vi "HostFormatPacket (1).vi"(11 "Enum in":u8) -> (3 "data string":string)   [LabVIEW 2017]
uses:
  Sensors/DataStreamIndex.ctl
  HostDataGLOBAL.vi
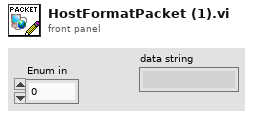
[diagram p1: front panel]
types:
  T1 = typedef "DataStreamIndex.ctl" = enum16{"SuspensionPT (PSI)", "MagBrakePT (PSI)", "Baby HPPT (PSI)", "BigRight HPPT (PSI)", "BigLeft HPPT (PSI)", "HallEffect FrontLeft (V)", "HallEffect FrontRight (V)", "HallEffect BackRight (V)", "HallEffect BackLeft (V)", "LinearPot FrontRight (V)", "LinearPot FrontLeft (V)", "LinearPot BackRight (V)", "LinearPot BackLeft (V)", "Speed (m/s)", "Distance (m)", "Piezo (V)", "Battery Voltage (V)", "Battery Current", "Battery Temperature (C)", "cRIO Temperature (C)", "Right Big Tank Temperature (C)", "Left Big Tank Temperature (C)", "Baby Tank Temperature (C)", "Right Manifold Temperature (C)", "Left Manifold Temperature (C)", "IMU Acceleration (m/s2)", "IMU Pressure (Pa)", "IMU Temperature (C)"}
  T2 = cluster{"Team ID":u8, "Enum in":u8, u32, u32, u32, u32, u32, u32, u32, u32}
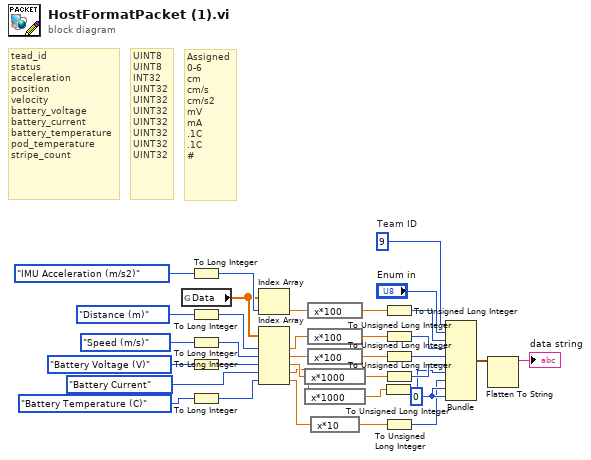
[diagram p0: block diagram]
diagram:
  w33 = u32 0
  w25 = u8 9  # Team ID
  # "Assigned\n0-6\ncm\ncm/s\ncm/s2\nmV\nmA\n.1C\n.1C\n#"
  # "UINT8\nUINT8\nINT32\nUINT32\nUINT32\nUINT32\nUINT32\nUINT32\nUINT32\nUINT32"
  # "tead_id\nstatus\nacceleration\nposition\nvelocity\nbattery_voltage\nbattery_current\nbattery_temperature\npod_temperature\nstripe_count"
  n1 = global read "HostDataGLOBAL.vi" "Data"() -> (w28:dbl[])
  n2 = To Long Integer(number=DataStreamIndex."IMU Acceleration (m/s2)" ("Data Stream Index")) -> (32bit integer=w29:i32)
  n3 = To Long Integer(number=DataStreamIndex."Distance (m)" ("Data Stream Index")) -> (32bit integer=w12:i32)
  n4 = To Long Integer(number=DataStreamIndex."Speed (m/s)" ("Data Stream Index")) -> (32bit integer=w26:i32)
  n5 = To Long Integer(number=DataStreamIndex."Battery Voltage (V)" ("Data Stream Index")) -> (32bit integer=w34:i32)
  n6 = To Long Integer(number=DataStreamIndex."Battery Temperature (C)" ("Data Stream Index")) -> (32bit integer=w7:i32)
  n7 = Index Array(array=w28, index=w29) -> (element=w27:dbl)
  n8 = Index Array(array=w28, index #1=w12, index #2=w26, index #3=w34, index #4=DataStreamIndex."Battery Current" ("Data Stream Index"), index #5=w7) -> (element #1=w11:dbl, element #2=w9:dbl, element #3=w35:dbl, element #4=w3:dbl, element #5=w4:dbl)
  n9 = expression code="x*1000"(w35) -> (w20:dbl)
  n10 = expression code="x*1000"(w3) -> (w2:dbl)
  n11 = expression code="x*100"(w27) -> (w17:dbl)
  n12 = expression code="x*100"(w11) -> (w15:dbl)
  n13 = expression code="x*100"(w9) -> (w10:dbl)
  n14 = expression code="x*10"(w4) -> (w22:dbl)
  n15 = To Unsigned Long Integer(number=w2) -> (unsigned 32bit integer=w1:u32)
  n16 = To Unsigned Long Integer(number=w17) -> (unsigned 32bit integer=w16:u32)
  n17 = To Unsigned Long Integer(number=w15) -> (unsigned 32bit integer=w18:u32)
  n18 = To Unsigned Long Integer(number=w10) -> (unsigned 32bit integer=w14:u32)
  n19 = To Unsigned Long Integer(number=w20) -> (unsigned 32bit integer=w19:u32)
  n20 = To Unsigned Long Integer(number=w22) -> (unsigned 32bit integer=w21:u32)
  n21 = Bundle("Team ID"=w25, "Enum in"="Enum in", w16, w18, w14, w19, w1, w21, w33, w33) -> (w24:T2)  [unwired: 1 in]
  n22 = Flatten To String(anything=w24) -> (data string=→"data string":string)  [unwired: 3 in, 2 out]
